vi "Insert Key Value Pair (String Array).vi"(7 "key":string, 8 "error in (no error)":errorcluster, 10 "JSON Data in":string[](array[string]), 11 "JSON Object in":refnum<class "JSON Object.lvclass">) -> (0 "error out":errorcluster, 1 "replaced":bool, 3 "JSON Object Out":refnum<class "JSON Object.lvclass">)   [LabVIEW 2015, in "LVJSON.lvlib" / "JSON Object.lvclass"]
uses:
  JSON Object.lvclass
  JSON Array/New JSON Array (String).vi
  Insert Key Value Pair (Single).vi
  JSON Helper/JSON Helper.lvclass
  JSON Array/JSON Array.lvclass
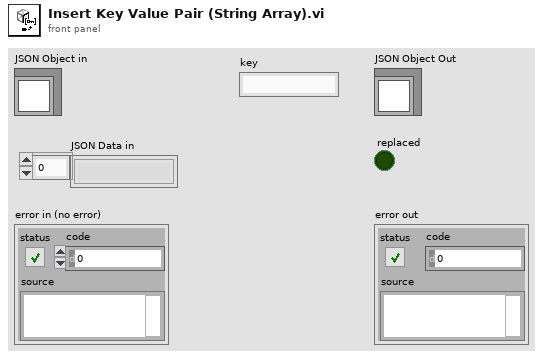
[diagram p1: front panel]
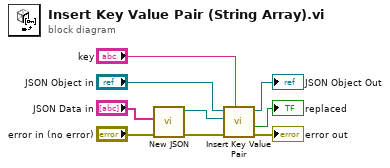
[diagram p0: block diagram]
diagram:
  n1 = call-poly "New JSON.vi"("error in (no error)"="error in (no error)", "String Array"="JSON Data in") -> ("error out"=w8:errorcluster, "JSON Array out"=w9:refnum<class "JSON Array.lvclass">)  [unwired: 8 in]
  n2 = call-poly "Insert Key Value Pair.vi"("key"="key", "error in (no error)"=w8, "value"=w9, "JSON Object in"="JSON Object in") -> ("error out"=→"error out":errorcluster, "replaced"=→"replaced":bool, "JSON Object out"=→"JSON Object Out":refnum<class "JSON Object.lvclass">)  [unwired: 5 in]
